vi "xcorr bkp normalized.vi"(4 "shift":u8, 6 "N":u8, 7 "y":u32, 8 "x":u32, 9 "enable":bool, 10 "lag":u16) -> (1 "Rxy valid":bool, 2 "Rxy":u64, 3 "trigger":bool)   [LabVIEW 2017]
uses:
  <vilib>/rvi/FXPMathLib/basic elements/FxpDiscreteDelay/XNode/nifxpmath_DiscreteDelay.xnode
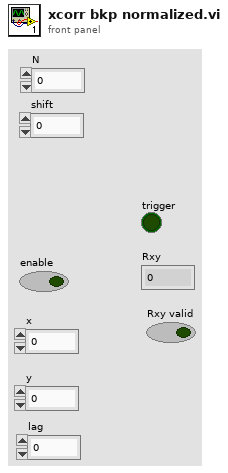
[diagram p1: front panel]
types:
  T1 = cluster{"Q":bool, "Q":bool, "Q":bool, "Q":bool, "valid":bool}
  T2 = cluster{"Q":bool, "Q":bool, "Q":bool, "Q":bool, "Q":bool, "Q":bool, "valid":bool}
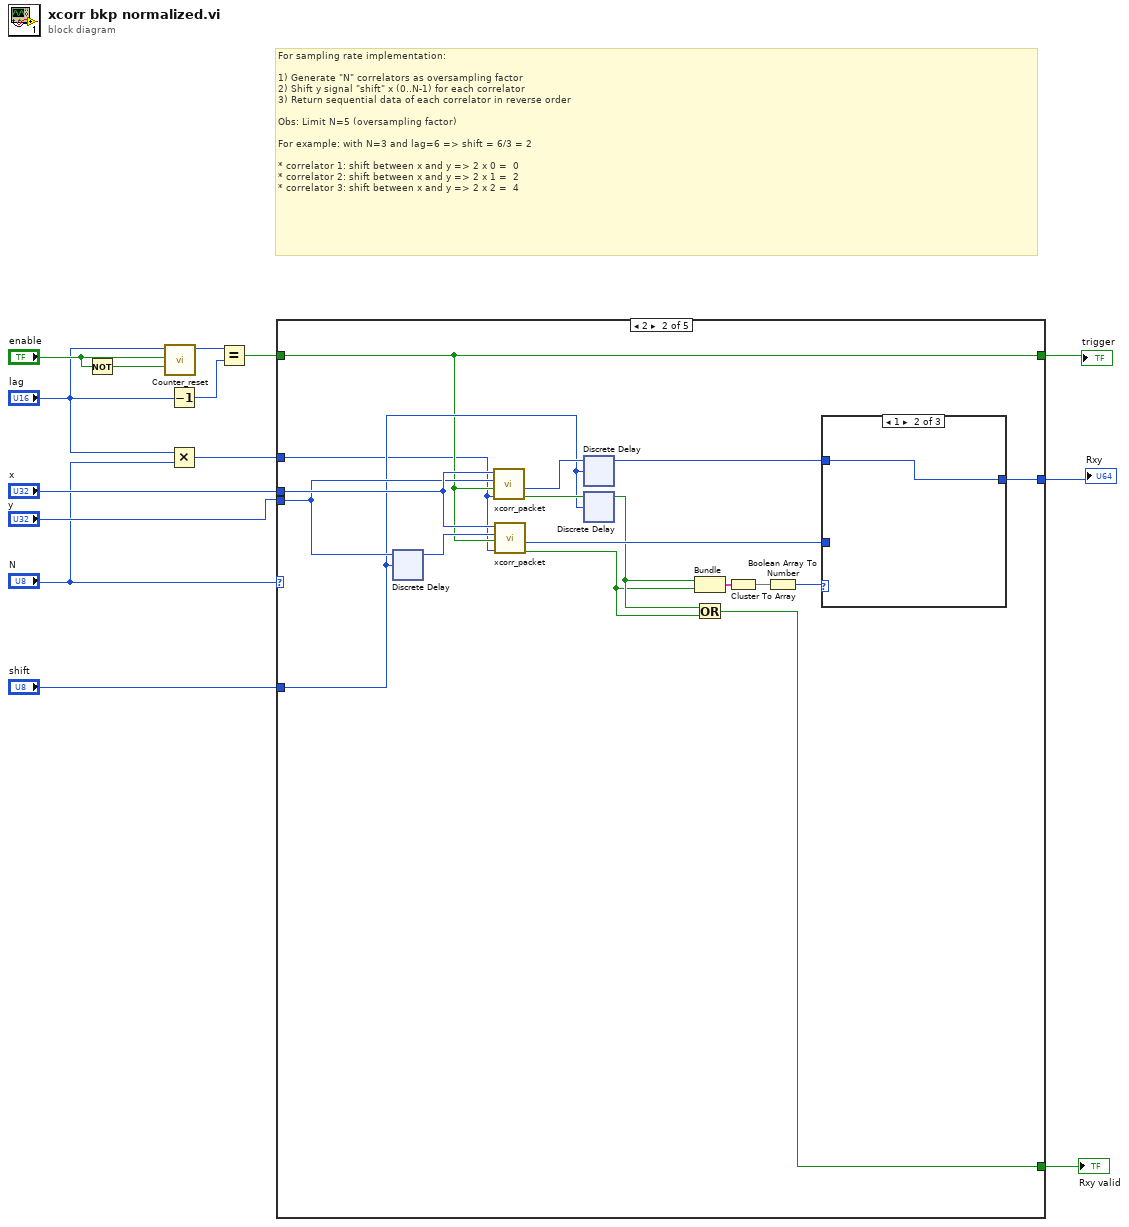
[diagram p0: block diagram]
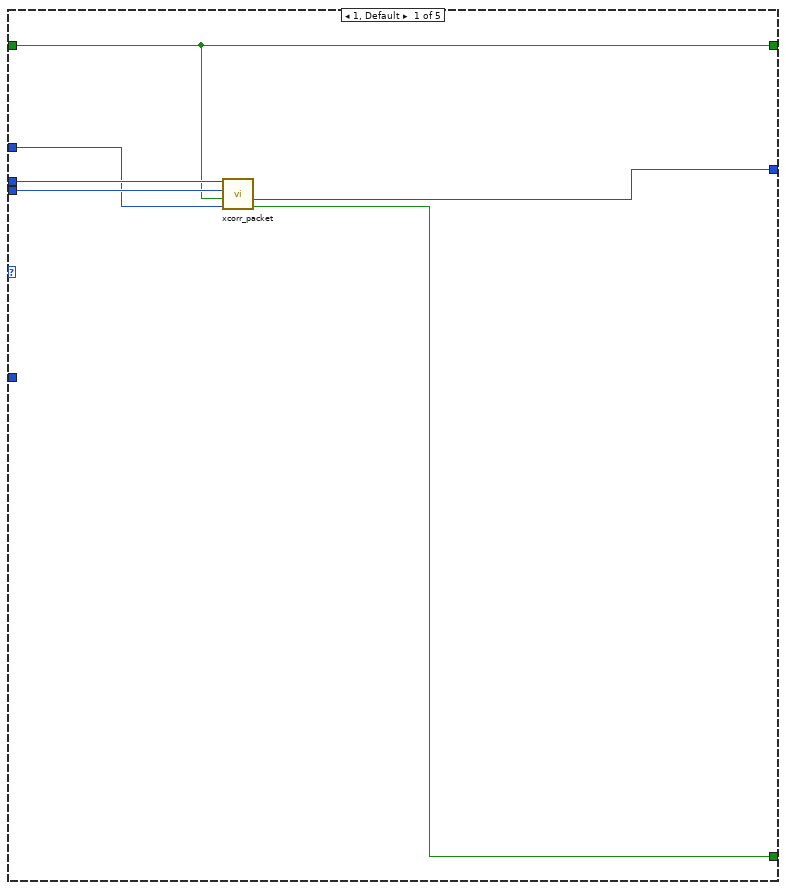
[diagram p2: hidden frame]
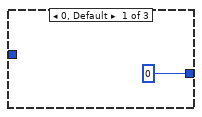
[diagram p3: hidden frame]
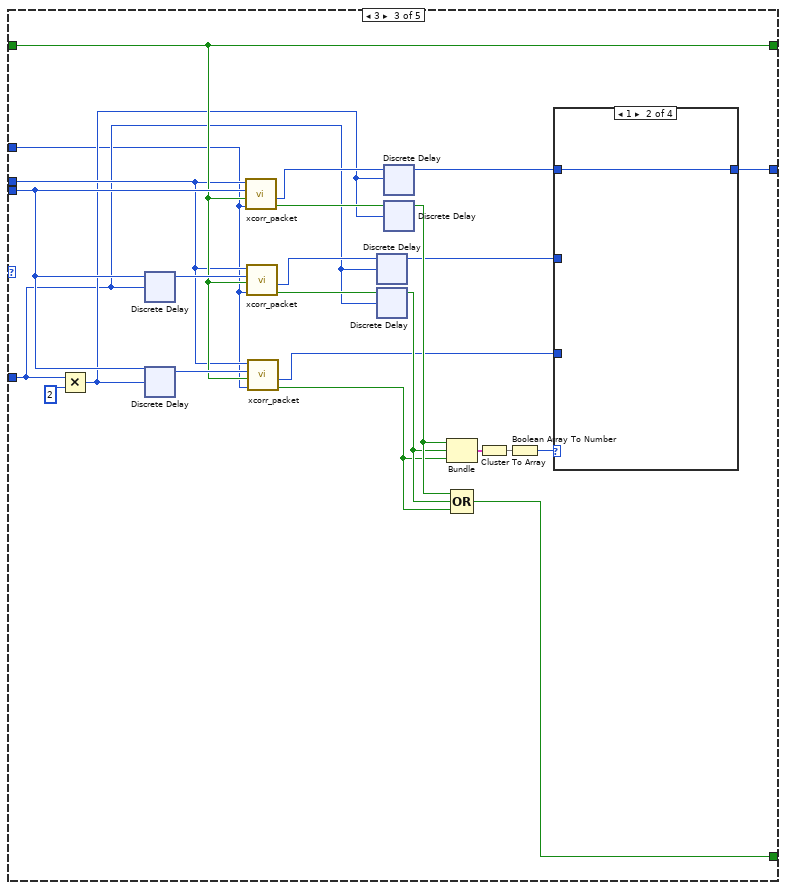
[diagram p5: hidden frame]
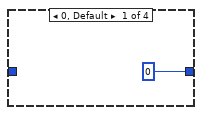
[diagram p6: hidden frame]
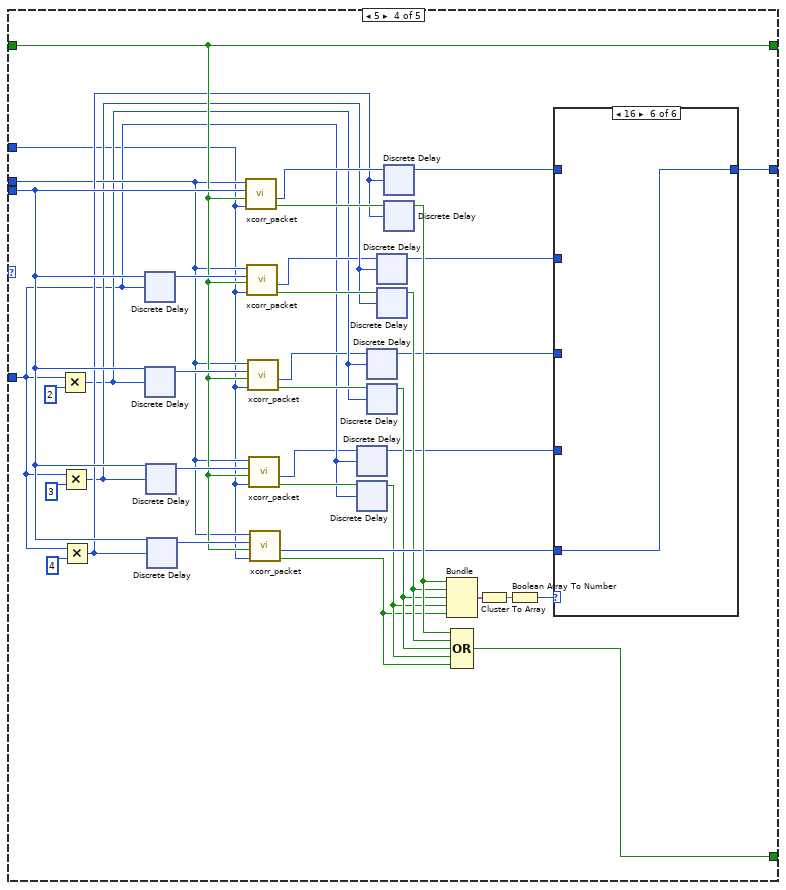
[diagram p9: hidden frame]
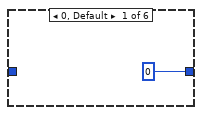
[diagram p10: hidden frame]
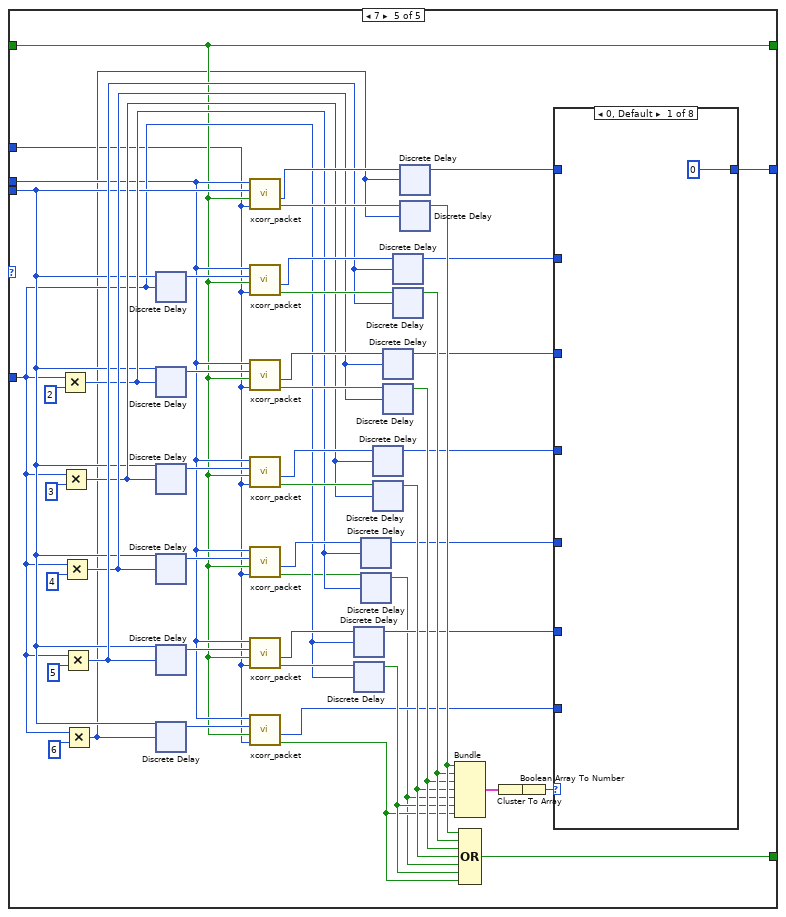
[diagram p15: hidden frame]
diagram:
  # "For sampling rate implementation:\n\n1) Generate \"N\" correlators as oversampling factor\n2) Shift y signal \"shift\" x (0..N-1) for each correlator\n3) Return sequential data of each correlator in reverse order\n\nObs: Limit N=5 (oversampling factor)\n\nFor example: with N=3 and lag=6 => shift = 6/3 = 2\n\n* correlator 1: shift between x and y => 2 x 0 =  0\n* correlator 2: shift between x and y => 2 x 1 =  2\n* correlator 3: shift between x and y => 2 x 2 =  4"
  n1 = Not(x="enable") -> (.not. x?=w10:bool)
  n2 = call "Counter_reset.vi"("reset"=w10, "enable"="enable", "limit"="lag") -> ("count"=w11:u16)  [unwired: 8 in]
  n3 = Decrement(x="lag") -> (x-1=w6:u16)
  n4 = Multiply(x="lag", y="N") -> (x*y=w1:u16)
  n5 = Equal?(x=w11, y=w6) -> (x = y?=w9:bool)
  n6 = case shown="2" "N" {
    tunnel: [w16 w24 w58 w98 w157] -> w4
    tunnel: [w20 w36 w64 w106 w164] -> w14
    tunnel: [w17 w30 w54 w90 w120] -> w13
    tunnel: w9 -> [w17 w30 w54 w90 w120]
    tunnel: "x" -> [w19 w37 w50 w80 w121]
    tunnel: "y" -> [w18 w35 w55 w91 w123]
    tunnel: "shift" -> [_ w31 w46 w72 w122]
    tunnel: w1 -> [w15 w21 w41 w69 w113]
    frame 1, Default {
      n7 = call "xcorr_packet.vi"("x"=w19, "y"=w18, "trigger"=w17, 3:w15) -> ("out"=w16:u64, "valid"=w20:bool)  [unwired: 4 in]
    }
    frame 2 {
      n8 = xnode ("Discrete Delay")("D"=w35, "n-1[0..255]"=w31) -> ("Q"=w34:u32)
      n9 = call "xcorr_packet.vi"("x"=w37, "y"=w35, "trigger"=w30, 3:w21) -> ("out"=w33:u64, "valid"=w32:bool)  [unwired: 4 in]
      n10 = call "xcorr_packet.vi"("x"=w37, "y"=w34, "trigger"=w30, 3:w21) -> ("out"=w25:u64, "valid"=w22:bool)  [unwired: 4 in]
      n11 = xnode ("Discrete Delay")("D"=w33, "n-1[0..255]"=w31) -> ("Q"=w26:u64)
      n12 = xnode ("Discrete Delay")("D"=w32, "n-1[0..255]"=w31) -> ("Q"=w23:bool)
      n13 = Bundle("Q"=w23, "valid"=w22) -> (w29:cluster{"Q":bool, "valid":bool})  [unwired: 1 in]
      n14 = Or(x=w23, y=w22) -> (x .or. y?=w36:bool)
      n15 = Cluster To Array(cluster=w29) -> (array=w28:bool[])
      n16 = Boolean Array To Number(Boolean array=w28) -> (number=w27:u8)
      n17 = case shown="1" w27 {
        tunnel: [u64 0 ("out") w39 w40] -> w24
        tunnel: w26 -> [_ w39 _]
        tunnel: w25 -> [_ _ w40]
        frame 0, Default {
        }
        frame 1 {
        }
        frame 2 {
        }
      }
    }
    frame 3 {
      n18 = Multiply(x=w46, y=u8 2 ("x")) -> (x*y=w47:u8)
      n19 = xnode ("Discrete Delay")("D"=w55, "n-1[0..255]"=w46) -> ("Q"=w63:u32)
      n20 = xnode ("Discrete Delay")("D"=w55, "n-1[0..255]"=w47) -> ("Q"=w56:u32)
      n21 = call "xcorr_packet.vi"("x"=w50, "y"=w55, "trigger"=w54, 3:w41) -> ("out"=w62:u64, "valid"=w61:bool)  [unwired: 4 in]
      n22 = call "xcorr_packet.vi"("x"=w50, "y"=w63, "trigger"=w54, 3:w41) -> ("out"=w49:u64, "valid"=w51:bool)  [unwired: 4 in]
      n23 = call "xcorr_packet.vi"("x"=w50, "y"=w56, "trigger"=w54, 3:w41) -> ("out"=w42:u64, "valid"=w43:bool)  [unwired: 4 in]
      n24 = xnode ("Discrete Delay")("D"=w49, "n-1[0..255]"=w46) -> ("Q"=w48:u64)
      n25 = xnode ("Discrete Delay")("D"=w51, "n-1[0..255]"=w46) -> ("Q"=w52:bool)
      n26 = xnode ("Discrete Delay")("D"=w62, "n-1[0..255]"=w47) -> ("Q"=w59:u64)
      n27 = xnode ("Discrete Delay")("D"=w61, "n-1[0..255]"=w47) -> ("Q"=w53:bool)
      n28 = Bundle("Q"=w53, "Q"=w52, "valid"=w43) -> (w45:cluster{"Q":bool, "Q":bool, "valid":bool})  [unwired: 1 in]
      n29 = Compound Arithmetic op=OR(w53, w52, w43) -> (w64:bool)
      n30 = Cluster To Array(cluster=w45) -> (array=w44:bool[])
      n31 = Boolean Array To Number(Boolean array=w44) -> (number=w60:u8)
      n32 = case shown="1" w60 {
        tunnel: [u64 0 ("out") w66 w67 w68] -> w58
        tunnel: w59 -> [_ w66 _ _]
        tunnel: w48 -> [_ _ w67 _]
        tunnel: w42 -> [_ _ _ w68]
        frame 0, Default {
        }
        frame 1 {
        }
        frame 2 {
        }
        frame 4 {
        }
      }
    }
    frame 5 {
      n33 = Multiply(x=w72, y=u8 2 ("x")) -> (x*y=w75:u8)
      n34 = Multiply(x=w72, y=u8 3 ("x")) -> (x*y=w78:u8)
      n35 = Multiply(x=w72, y=u8 4 ("x")) -> (x*y=w87:u8)
      n36 = xnode ("Discrete Delay")("D"=w91, "n-1[0..255]"=w72) -> ("Q"=w105:u32)
      n37 = xnode ("Discrete Delay")("D"=w91, "n-1[0..255]"=w75) -> ("Q"=w96:u32)
      n38 = xnode ("Discrete Delay")("D"=w91, "n-1[0..255]"=w78) -> ("Q"=w94:u32)
      n39 = xnode ("Discrete Delay")("D"=w91, "n-1[0..255]"=w87) -> ("Q"=w92:u32)
      n40 = call "xcorr_packet.vi"("x"=w80, "y"=w91, "trigger"=w90, 3:w69) -> ("out"=w104:u64, "valid"=w103:bool)  [unwired: 4 in]
      n41 = call "xcorr_packet.vi"("x"=w80, "y"=w105, "trigger"=w90, 3:w69) -> ("out"=w77:u64, "valid"=w85:bool)  [unwired: 4 in]
      n42 = call "xcorr_packet.vi"("x"=w80, "y"=w96, "trigger"=w90, 3:w69) -> ("out"=w74:u64, "valid"=w84:bool)  [unwired: 4 in]
      n43 = call "xcorr_packet.vi"("x"=w80, "y"=w94, "trigger"=w90, 3:w69) -> ("out"=w71:u64, "valid"=w82:bool)  [unwired: 4 in]
      n44 = call "xcorr_packet.vi"("x"=w80, "y"=w92, "trigger"=w90, 3:w69) -> ("out"=w88:u64, "valid"=w79:bool)  [unwired: 4 in]
      n45 = xnode ("Discrete Delay")("D"=w71, "n-1[0..255]"=w72) -> ("Q"=w70:u64)
      n46 = xnode ("Discrete Delay")("D"=w82, "n-1[0..255]"=w72) -> ("Q"=w81:bool)
      n47 = xnode ("Discrete Delay")("D"=w74, "n-1[0..255]"=w75) -> ("Q"=w73:u64)
      n48 = xnode ("Discrete Delay")("D"=w84, "n-1[0..255]"=w75) -> ("Q"=w83:bool)
      n49 = xnode ("Discrete Delay")("D"=w77, "n-1[0..255]"=w78) -> ("Q"=w76:u64)
      n50 = xnode ("Discrete Delay")("D"=w85, "n-1[0..255]"=w78) -> ("Q"=w86:bool)
      n51 = xnode ("Discrete Delay")("D"=w104, "n-1[0..255]"=w87) -> ("Q"=w99:u64)
      n52 = xnode ("Discrete Delay")("D"=w103, "n-1[0..255]"=w87) -> ("Q"=w89:bool)
      n53 = Bundle("Q"=w89, "Q"=w86, "Q"=w83, "Q"=w81, "valid"=w79) -> (w102:T1)  [unwired: 1 in]
      n54 = Compound Arithmetic op=OR(w89, w86, w83, w81, w79) -> (w106:bool)
      n55 = Cluster To Array(cluster=w102) -> (array=w101:bool[])
      n56 = Boolean Array To Number(Boolean array=w101) -> (number=w100:u8)
      n57 = case shown="16" w100 {
        tunnel: [u64 0 ("out") w108 w109 w110 w111 w112] -> w98
        tunnel: w99 -> [_ w108 _ _ _ _]
        tunnel: w76 -> [_ _ w109 _ _ _]
        tunnel: w73 -> [_ _ _ w110 _ _]
        tunnel: w70 -> [_ _ _ _ w111 _]
        tunnel: w88 -> [_ _ _ _ _ w112]
        frame 0, Default {
        }
        frame 1 {
        }
        frame 2 {
        }
        frame 4 {
        }
        frame 8 {
        }
        frame 16 {
        }
      }
    }
    frame 7 {
      n58 = Multiply(x=w122, y=u8 2 ("x")) -> (x*y=w126:u8)
      n59 = Multiply(x=w122, y=u8 3 ("x")) -> (x*y=w127:u8)
      n60 = Multiply(x=w122, y=u8 4 ("x")) -> (x*y=w128:u8)
      n61 = Multiply(x=w122, y=u8 5 ("x")) -> (x*y=w129:u8)
      n62 = Multiply(x=w122, y=u8 6 ("x")) -> (x*y=w117:u8)
      n63 = xnode ("Discrete Delay")("D"=w123, "n-1[0..255]"=w122) -> ("Q"=w163:u32)
      n64 = xnode ("Discrete Delay")("D"=w123, "n-1[0..255]"=w126) -> ("Q"=w155:u32)
      n65 = xnode ("Discrete Delay")("D"=w123, "n-1[0..255]"=w127) -> ("Q"=w153:u32)
      n66 = xnode ("Discrete Delay")("D"=w123, "n-1[0..255]"=w128) -> ("Q"=w151:u32)
      n67 = xnode ("Discrete Delay")("D"=w123, "n-1[0..255]"=w129) -> ("Q"=w136:u32)
      n68 = xnode ("Discrete Delay")("D"=w123, "n-1[0..255]"=w117) -> ("Q"=w124:u32)
      n69 = call "xcorr_packet.vi"("x"=w121, "y"=w123, "trigger"=w120, 3:w113) -> ("out"=w162:u64, "valid"=w161:bool)  [unwired: 4 in]
      n70 = call "xcorr_packet.vi"("x"=w121, "y"=w163, "trigger"=w120, 3:w113) -> ("out"=w143:u64, "valid"=w148:bool)  [unwired: 4 in]
      n71 = call "xcorr_packet.vi"("x"=w121, "y"=w155, "trigger"=w120, 3:w113) -> ("out"=w141:u64, "valid"=w147:bool)  [unwired: 4 in]
      n72 = call "xcorr_packet.vi"("x"=w121, "y"=w153, "trigger"=w120, 3:w113) -> ("out"=w139:u64, "valid"=w145:bool)  [unwired: 4 in]
      n73 = call "xcorr_packet.vi"("x"=w121, "y"=w151, "trigger"=w120, 3:w113) -> ("out"=w131:u64, "valid"=w115:bool)  [unwired: 4 in]
      n74 = call "xcorr_packet.vi"("x"=w121, "y"=w136, "trigger"=w120, 3:w113) -> ("out"=w133:u64, "valid"=w135:bool)  [unwired: 4 in]
      n75 = call "xcorr_packet.vi"("x"=w121, "y"=w124, "trigger"=w120, 3:w113) -> ("out"=w116:u64, "valid"=w119:bool)  [unwired: 4 in]
      n76 = xnode ("Discrete Delay")("D"=w133, "n-1[0..255]"=w122) -> ("Q"=w132:u64)
      n77 = xnode ("Discrete Delay")("D"=w135, "n-1[0..255]"=w122) -> ("Q"=w134:bool)
      n78 = xnode ("Discrete Delay")("D"=w131, "n-1[0..255]"=w126) -> ("Q"=w130:u64)
      n79 = xnode ("Discrete Delay")("D"=w115, "n-1[0..255]"=w126) -> ("Q"=w114:bool)
      n80 = xnode ("Discrete Delay")("D"=w139, "n-1[0..255]"=w127) -> ("Q"=w138:u64)
      n81 = xnode ("Discrete Delay")("D"=w145, "n-1[0..255]"=w127) -> ("Q"=w144:bool)
      n82 = xnode ("Discrete Delay")("D"=w141, "n-1[0..255]"=w128) -> ("Q"=w140:u64)
      n83 = xnode ("Discrete Delay")("D"=w147, "n-1[0..255]"=w128) -> ("Q"=w146:bool)
      n84 = xnode ("Discrete Delay")("D"=w143, "n-1[0..255]"=w129) -> ("Q"=w142:u64)
      n85 = xnode ("Discrete Delay")("D"=w148, "n-1[0..255]"=w129) -> ("Q"=w149:bool)
      n86 = xnode ("Discrete Delay")("D"=w162, "n-1[0..255]"=w117) -> ("Q"=w158:u64)
      n87 = xnode ("Discrete Delay")("D"=w161, "n-1[0..255]"=w117) -> ("Q"=w150:bool)
      n88 = Bundle("Q"=w150, "Q"=w149, "Q"=w146, "Q"=w144, "Q"=w114, "Q"=w134, "valid"=w119) -> (w118:T2)  [unwired: 1 in]
      n89 = Compound Arithmetic op=OR(w150, w149, w146, w144, w114, w134, w119) -> (w164:bool)
      n90 = Cluster To Array(cluster=w118) -> (array=w160:bool[])
      n91 = Boolean Array To Number(Boolean array=w160) -> (number=w159:u8)
      n92 = case shown="0, Default" w159 {
        tunnel: [u64 0 ("out") w166 w167 w168 w169 w170 w171 w172] -> w157
        tunnel: w158 -> [_ w166 _ _ _ _ _ _]
        tunnel: w142 -> [_ _ w167 _ _ _ _ _]
        tunnel: w140 -> [_ _ _ w168 _ _ _ _]
        tunnel: w138 -> [_ _ _ _ w169 _ _ _]
        tunnel: w130 -> [_ _ _ _ _ w170 _ _]
        tunnel: w132 -> [_ _ _ _ _ _ w171 _]
        tunnel: w116 -> [_ _ _ _ _ _ _ w172]
        frame 0, Default {
        }
        frame 1 {
        }
        frame 2 {
        }
        frame 4 {
        }
        frame 8 {
        }
        frame 16 {
        }
        frame 32 {
        }
        frame 64 {
        }
      }
    }
  }
  "trigger" <- w13
  "Rxy valid" <- w14
  "Rxy" <- w4
